vi "Сохранение графика.vi"(11 "String":string) -> ()   [LabVIEW 2011]
panel:
  out "т1 2":waveform(dbl)[](graph)
  out "т1":waveform(dbl)[](graph)
  in  "Сохранить":bool
  # "С1"
  # "С2"
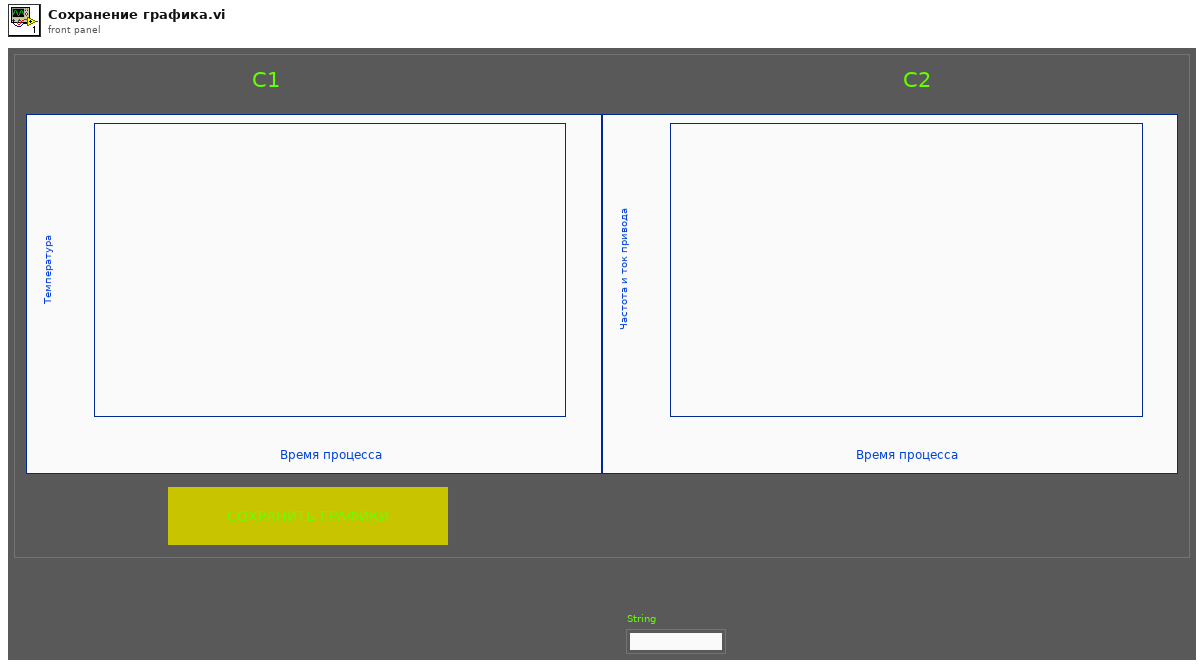
[diagram p1: front panel]
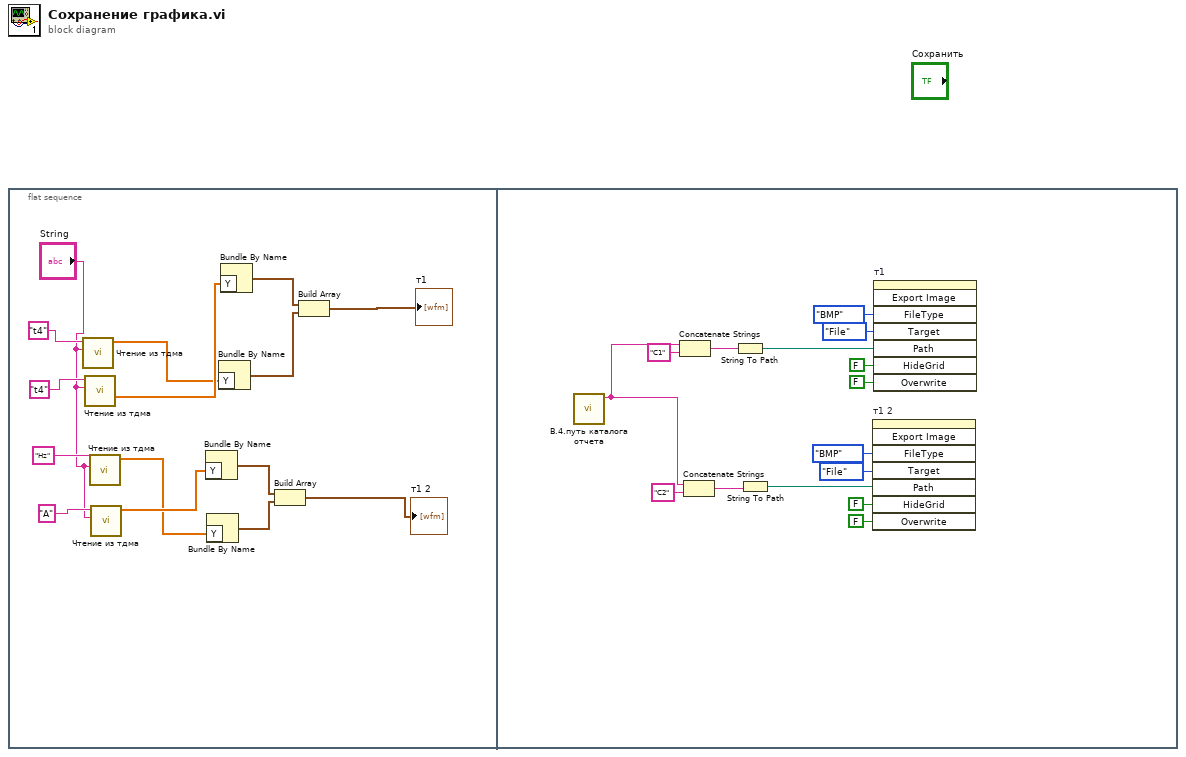
[diagram p0: block diagram]
diagram:
  n1 = flat-sequence {
    frame #0 {
      n2 = call "Чтение из тдма.vi"("tdm"="String", "Канал"="t4") -> ("data"=w2:dbl[])  [unwired: 9 in]
      n3 = call "Чтение из тдма.vi"("tdm"="String", "Канал"="t4") -> ("data"=w3:dbl[])  [unwired: 9 in]
      n4 = call "Чтение из тдма.vi"("tdm"="String", "Канал"="Hz") -> ("data"=w4:dbl[])  [unwired: 9 in]
      n5 = call "Чтение из тдма.vi"("tdm"="String", "Канал"="A") -> ("data"=w5:dbl[])  [unwired: 9 in]
      n6 = Bundle By Name("Y"=w5) -> (w7:waveform(dbl))  [unwired: 1 in]
      n7 = Bundle By Name("Y"=w4) -> (w8:waveform(dbl))  [unwired: 1 in]
      n8 = Bundle By Name("Y"=w2) -> (w12:waveform(dbl))  [unwired: 1 in]
      n9 = Bundle By Name("Y"=w3) -> (w13:waveform(dbl))  [unwired: 1 in]
      n10 = Build Array(w7, w8) -> (→"т1 2":waveform(dbl)[])
      n11 = Build Array(w13, w12) -> (→"т1":waveform(dbl)[])
    }
    frame #1 {
      n12 = call "B.4.путь каталога отчета.vi"() -> ("path_out"=w28:string)  [unwired: 11 in]
      n13 = Concatenate Strings(w28, "C1" ("string")) -> (w26:string)
      n14 = Concatenate Strings(w28, "C2" ("string")) -> (w24:string)
      n15 = String To Path(string=w26) -> (path=w27:path)
      n16 = String To Path(string=w24) -> (path=w25:path)
      n17 = invoke on="т1 2" class="WFGraph (strict)" method="Export Image"("FileType"=enum32{"BMP", "EPS", "EMF", "PICT"}."BMP" ("File Type"), "Target"=enum32{"File", "Clipboard"}."File", "Path"=w25, "HideGrid"=FALSE ("Hide Grid"), "Overwrite"=FALSE ("Always Overwrite")) -> ()  [unwired: 3 in, 8 out]
      n18 = invoke on="т1" class="WFGraph (strict)" method="Export Image"("FileType"=enum32{"BMP", "EPS", "EMF", "PICT"}."BMP" ("File Type"), "Target"=enum32{"File", "Clipboard"}."File", "Path"=w27, "HideGrid"=FALSE ("Hide Grid"), "Overwrite"=FALSE ("Always Overwrite")) -> ()  [unwired: 3 in, 8 out]
    }
  }
